vi "CalculateTrialPerformance.vi"(6 "nGoTrials":i16, 7 "nTrials":i32, 8 "nFalseAlarms":i32, 9 "nMiss":i32, 10 "nCorrect Rejections":i32, 11 "nHits":i32) -> (2 "pCorrect":dbl, 3 "D'prime":dbl)   [LabVIEW 2013]
uses:
  <vilib>/gmath/statdist.llb/Normal Inverse CDF.vi
  <vilib>/gmath/NI_Gmath.lvlib
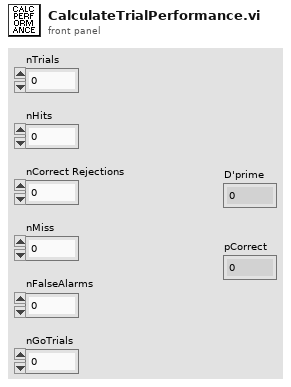
[diagram p1: front panel]
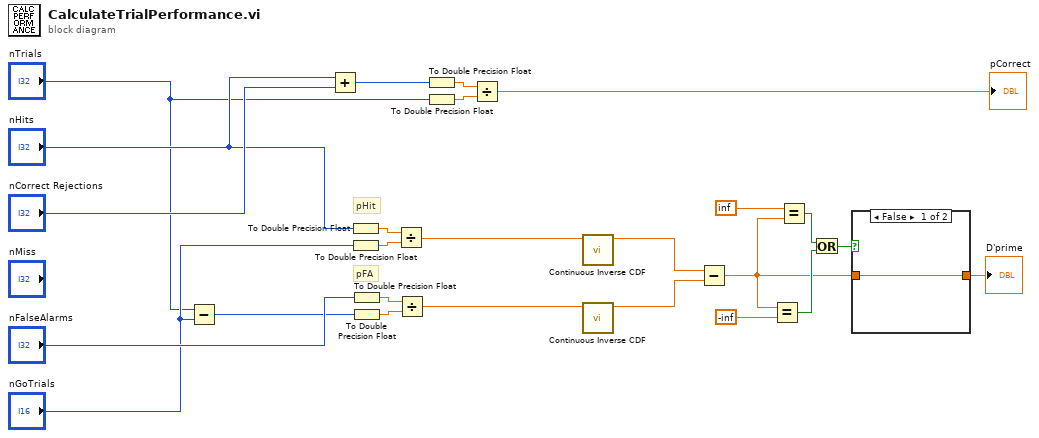
[diagram p0: block diagram]
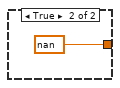
[diagram p2: hidden frame]
diagram:
  # "pFA"
  # "pHit"
  n1 = Subtract(x="nTrials", y="nGoTrials") -> (x-y=w19:i32)
  n2 = Add(x="nHits", y="nCorrect Rejections") -> (x+y=w10:i32)
  n3 = To Double Precision Float(number="nHits") -> (double precision float=w25:dbl)
  n4 = To Double Precision Float(number="nGoTrials") -> (double precision float=w24:dbl)
  n5 = To Double Precision Float(number="nFalseAlarms") -> (double precision float=w22:dbl)
  n6 = To Double Precision Float(number=w19) -> (double precision float=w23:dbl)
  n7 = Divide(x=w25, y=w24) -> (x/y=w17:dbl)
  n8 = Divide(x=w22, y=w23) -> (x/y=w18:dbl)
  n9 = To Double Precision Float(number=w10) -> (double precision float=w11:dbl)
  n10 = To Double Precision Float(number="nTrials") -> (double precision float=w12:dbl)
  n11 = Divide(x=w11, y=w12) -> (x/y=→"pCorrect":dbl)
  n12 = call-poly <vilib>:"Continuous Inverse CDF.vi"("cdf(x)"=w17) -> ("x"=w16:dbl)  [unwired: 9 in, 1 out]
  n13 = call-poly <vilib>:"Continuous Inverse CDF.vi"("cdf(x)"=w18) -> ("x"=w15:dbl)  [unwired: 9 in, 1 out]
  n14 = Subtract(x=w16, y=w15) -> (x-y=w1:dbl)
  n15 = Equal?(x=w1, y=-inf) -> (x = y?=w5:bool)
  n16 = Equal?(x=inf, y=w1) -> (x = y?=w4:bool)
  n17 = Or(x=w4, y=w5) -> (x .or. y?=w3:bool)
  n18 = case shown="False" w3 {
    tunnel: [w26 nan] -> w2
    tunnel: w1 -> [w26 _]
    frame False {
    }
    frame True {
    }
  }
  "D'prime" <- w2
